vi "Do.vi"(8 "error in (no error)":errorcluster, 9 "CommandQueueIn":refnum<queue>, 10 "DataNotifierIn":refnum<notifier>, 11 "CommandCopy in":refnum<class "Display.lvclass">) -> (0 "error out":errorcluster, 1 "ExitFlag":bool, 2 "DataNotifierOut":refnum<notifier>, 3 "CommandCopy out":refnum<class "Display.lvclass">)   [LabVIEW 2013, in "Display.lvclass"]
uses:
  Display.lvclass
  SystemData.lvclass/SystemData.lvclass
  RootCommand.lvclass/RootCommand.lvclass
  SystemData.lvclass/SystemData.lvclass/SystemData.ctl
  Generator.lvclass/Generator.lvclass
panel:
  # "notifier包裝SystemData物件的參考"
  # "命令物件序列參考"
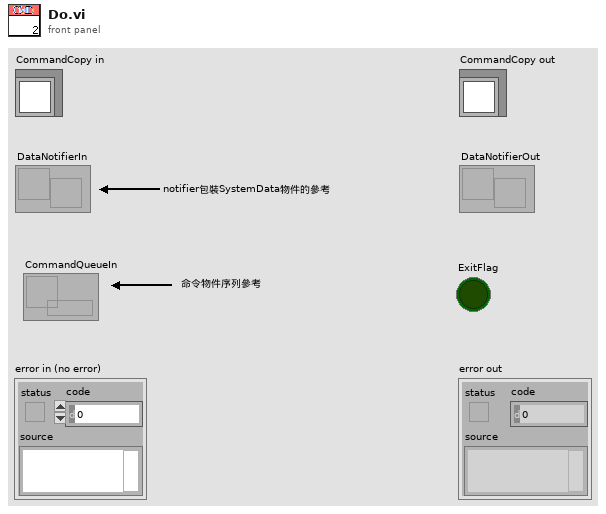
[diagram p1: front panel]
types:
  T1 = typedef "SystemData.lvclass/SystemDataTypeDefine.ctl" = cluster{"ThisVIParameter":cluster{"ThisVIPath":path, "ThisVIReference":refnum<vi>, "AllControlReference":refnum<vi>[]}, "GeneratorParameter":cluster{"Frequency":dbl, "Amplitude":dbl}, "WaveformBuffer":waveform(dbl), "SourceSelect":u16, "GeneratorClassArray":refnum<class "Generator.lvclass">[]}
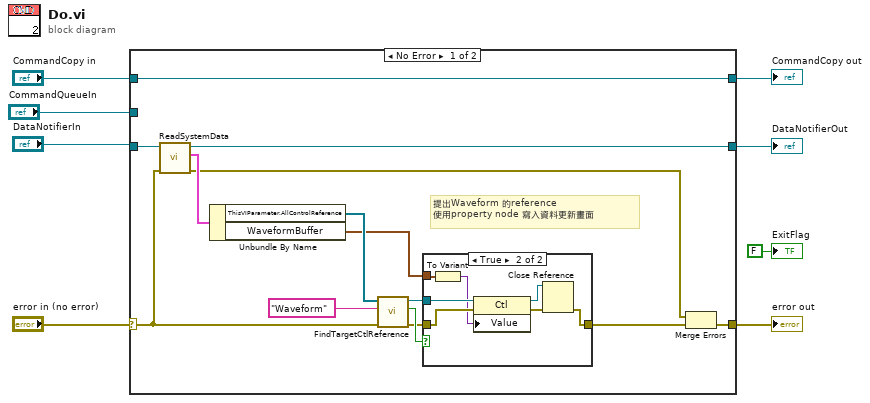
[diagram p0: block diagram]
diagram:
  n1 = case shown="No Error" "error in (no error)" {
    selector: "error in (no error)" -> [w19 w33]
    tunnel: [w18 w33] -> w4
    tunnel: [w22 w32] -> w3
    tunnel: "CommandCopy in" -> [w22 w32]
    tunnel: "DataNotifierIn" -> [w21 w31]
    tunnel: [w10 w31] -> w2
    tunnel: "CommandQueueIn" -> [_ _]
    frame No Error {
      # "提出Waveform 的reference\n使用property node 寫入資料更新畫面"
      n2 = call "ReadSystemData.vi"("error in (no error)"=w19, "DataNotifierIn"=w21) -> ("error out"=w9:errorcluster, "SystemData"=w20:T1, "DataNotifierIn"=w10:refnum<notifier>)  [unwired: 7 in]
      n3 = Unbundle By Name(w20) -> ("ThisVIParameter.AllControlReference"=w16:refnum<vi>[], "WaveformBuffer"=w11:waveform(dbl))
      n4 = call "FindTargetCtlReference.vi"("error in (no error)"=w19, "TargetCtlLabel.Text"="Waveform", "AllControlReference"=w16) -> ("error out"=w12:errorcluster, "Find?"=w14:bool, "TargetCtlRefnum"=w13:refnum<vi>)  [unwired: 6 in]
      n5 = case shown="True" w14 {
        tunnel: w13 -> [_ w30]
        tunnel: w12 -> [w23 w29]
        tunnel: w11 -> [_ w27]
        tunnel: [w23 w25] -> w17
        frame False {
        }
        frame True {
          n6 = To Variant(anything=w27) -> (Variant=w28:variant)
          n7 = property class="Ctl"(reference=w30, error in=w29, "Value"=w28) -> (reference out=w24:refnum<vi>, error out=w26:errorcluster)
          n8 = Close Reference(reference=w24, error in (no error)=w26) -> (error out=w25:errorcluster)
        }
      }
      n9 = Merge Errors(w9, w17) -> (w18:errorcluster)
    }
    frame Error {
    }
  }
  "error out" <- w4
  "CommandCopy out" <- w3
  "DataNotifierOut" <- w2
  "ExitFlag" <- FALSE ("ExitFlag")
